vi "Ev Key Down.vi"(8 "error in (no error)":errorcluster, 9 "PlatMods":T1, 10 "Char":i16, 11 "LF2R IDE in":refnum<class "Main Panel.lvclass">) -> (0 "error out":errorcluster, 3 "LF2R IDE out":refnum<class "Main Panel.lvclass">)   [LabVIEW 2018, in "Main Panel.lvlib" / "Main Panel.lvclass"]
uses:
  Main Panel.lvclass
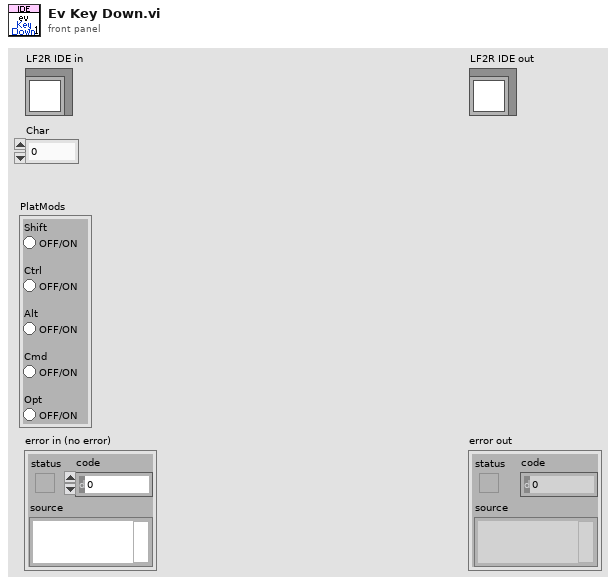
[diagram p1: front panel]
types:
  T1 = cluster{"Shift":bool, "Ctrl":bool, "Alt":bool, "Cmd":bool, "Opt":bool}
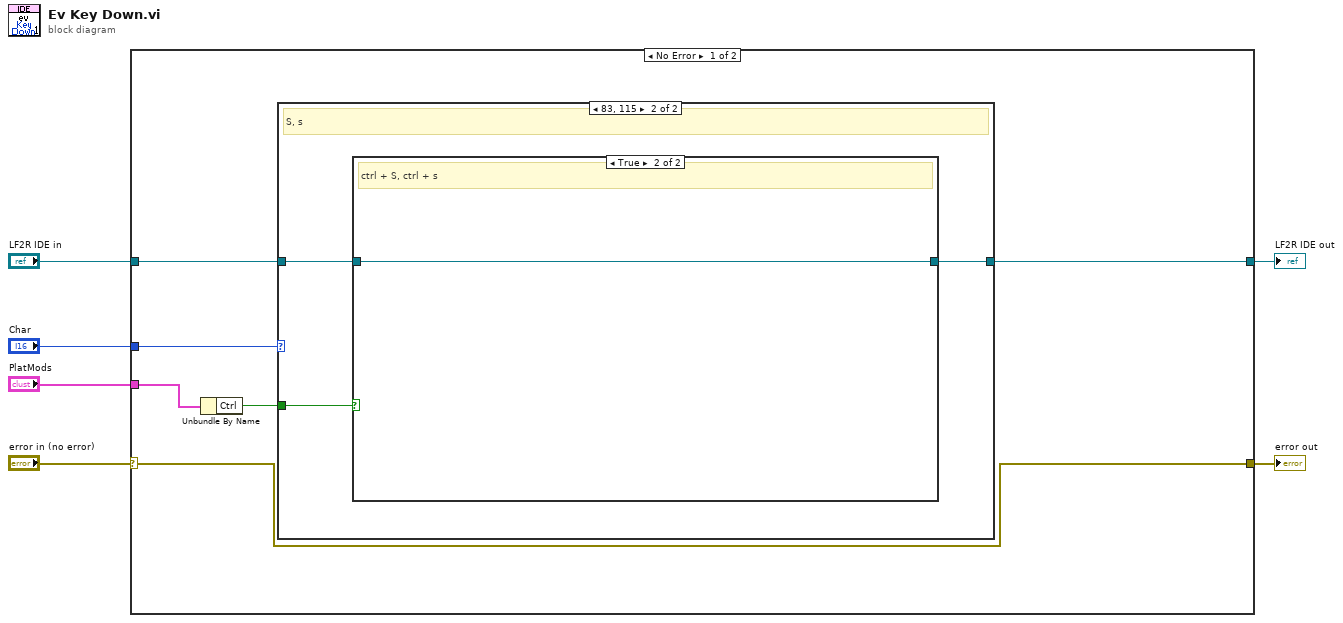
[diagram p0: block diagram]
diagram:
  n1 = case shown="No Error" "error in (no error)" {
    selector: "error in (no error)" -> [w7 w20]
    tunnel: [w7 w20] -> w5
    tunnel: [w8 w19] -> w3
    tunnel: "LF2R IDE in" -> [w9 w19]
    tunnel: "Char" -> [w12 _]
    tunnel: "PlatMods" -> [w11 _]
    frame No Error {
      n2 = Unbundle By Name(w11) -> ("Ctrl"=w10:bool)
      n3 = case shown="83, 115" w12 {
        tunnel: w10 -> [_ w16]
        tunnel: w9 -> [w13 w15]
        tunnel: [w13 w14] -> w8
        frame 0, Default {
        }
        frame 83, 115 {
          # "S, s"
          n4 = case shown="True" w16 {
            tunnel: w15 -> [w17 w18]
            tunnel: [w17 w18] -> w14
            frame False {
            }
            frame True {
              # "ctrl + S, ctrl + s"
            }
          }
        }
      }
    }
    frame Error {
    }
  }
  "error out" <- w5
  "LF2R IDE out" <- w3
